vi "AttackerStop.vi"(6 "atacando contra?":bool, 8 "IA State Input 2":T1, 9 "balls":T5[](array[typedef]), 10 "Field Size in":T6, 11 "Robot in":T2={"id"=0, "function"=enum."Attacker", "x"=0.0, "y"=0.0, "orientation"=0.0, "v_tangent"=0.0, "v_normal"=0.0, "v_ang"=0.0, "kick_x"=0.0, "kick_z"=0.0, "dribble"=FALSE, "Timestamp"=timestamp(0 s since 1904-01-01), "dest_x"=0.0, "dest_y"=0.0, "dest_orientation"=0.0, "estimatives"={"est_v_tangent"=0.0, "est_v_normal"=0.0, "est_vx"=0.0, "est_vy"=0.0}, "dest_x_kick"=0.0, "dest_y_kick"=0.0, "Gap Coord"=[], "States"=enum."GoToTangent"}) -> (3 "Robot out":T2={"id"=0, "function"=enum."Attacker", "x"=0.0, "y"=0.0, "orientation"=0.0, "v_tangent"=0.0, "v_normal"=0.0, "v_ang"=0.0, "kick_x"=0.0, "kick_z"=0.0, "dribble"=FALSE, "Timestamp"=timestamp(0 s since 1904-01-01), "dest_x"=0.0, "dest_y"=0.0, "dest_orientation"=0.0, "estimatives"={"est_v_tangent"=0.0, "est_v_normal"=0.0, "est_vx"=0.0, "est_vy"=0.0}, "dest_x_kick"=0.0, "dest_y_kick"=0.0, "Gap Coord"=[], "States"=enum."GoToTangent"})   [LabVIEW 2016]
uses:
  Core/Field Size.ctl
  Core/AI Robot.ctl
  Functions Enum.ctl
  AttackerStates.ctl
  Core/AI Ball.ctl
  Core/AI Input.ctl
  Core/AI Judge.ctl
  Command Enum.ctl
  Util/Events/Events.ctl
  <vilib>/Analysis/_algsub.llb/Real Vector Norm.vi
  <vilib>/Analysis/NI_AALPro.lvlib
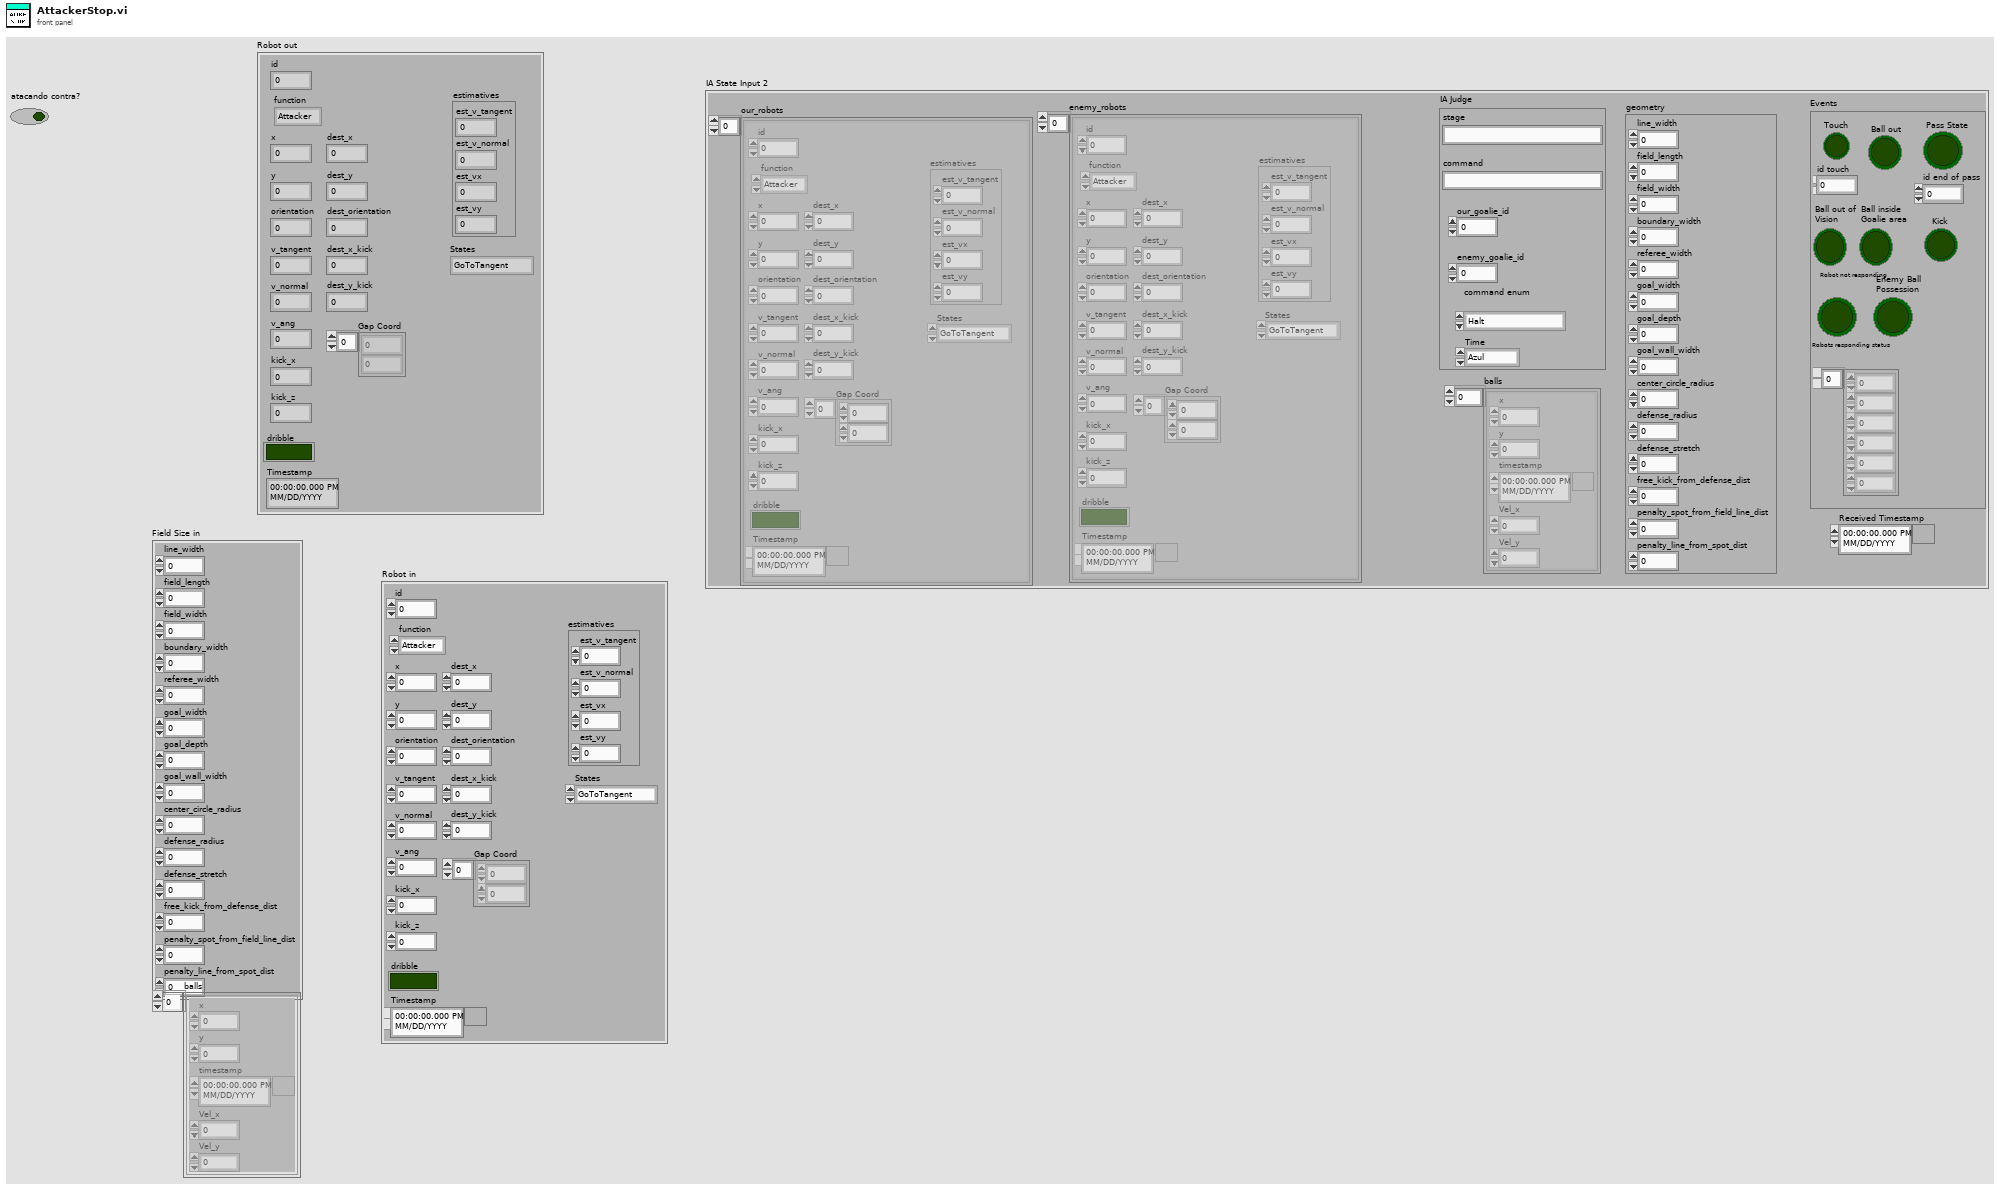
[diagram p1: front panel]
types:
  T1 = typedef "AI Input.ctl" = cluster{"our_robots":T2[], "enemy_robots":T2[], "balls":T5[], "geometry":T6, "IA Judge":T7, "Received Timestamp":timestamp, "Events":T9}
  T2 = typedef "AI Robot.ctl" = cluster{"id":u32, "function":T3, "x":dbl, "y":dbl, "orientation":dbl, "v_tangent":dbl, "v_normal":dbl, "v_ang":dbl, "kick_x":dbl, "kick_z":dbl, "dribble":bool, "Timestamp":timestamp, "dest_x":dbl, "dest_y":dbl, "dest_orientation":dbl, "estimatives":cluster{"est_v_tangent":dbl, "est_v_normal":dbl, "est_vx":dbl, "est_vy":dbl}, "dest_x_kick":dbl, "dest_y_kick":dbl, "Gap Coord":dbl[], "States":T4}
  T3 = typedef "Functions Enum.ctl" = enum16{"Attacker", "Goalie", "Defender", "Striker", "Goto 0", "Dummy", "Kicker", "ZigZag"}
  T4 = typedef "AttackerStates.ctl" = enum16{"Pass", "GoToTangent", "BallGetting", "GoToKick", ""}
  T5 = typedef "AI Ball.ctl" = cluster{"x":dbl, "y":dbl, "timestamp":timestamp, "Vel_x":dbl, "Vel_y":dbl}
  T6 = typedef "Field Size.ctl" = cluster{"line_width":u32, "field_length":u32, "field_width":u32, "boundary_width":u32, "referee_width":u32, "goal_width":u32, "goal_depth":u32, "goal_wall_width":u32, "center_circle_radius":u32, "defense_radius":u32, "defense_stretch":u32, "free_kick_from_defense_dist":u32, "penalty_spot_from_field_line_dist":u32, "penalty_line_from_spot_dist":u32}
  T7 = typedef "AI Judge.ctl" = cluster{"stage":string, "command":string, "our_goalie_id":dbl, "enemy_goalie_id":dbl, "command enum":T8, "Time":enum16{"Azul", "Amarelo"}}
  T8 = typedef "Command Enum.ctl" = enum16{"Halt", "Stop", "Force Start", "PKA Normal Start", "Prepare Kickoff Ally", "PKE Normal Start", "Prepare Kickoff Enemy", "Prepare Penalty Ally", "PPA Normal Start", "Prepare Penalty Enemy", "PPE Normal Start", "Direct Free Enemy", "Direct Free Ally", "Indirect Free Enemy", "Indirect Free Ally", "Timeout Enemy", "Timeout Ally", "Goal Enemy", "Goal Ally", "Ball Placement Enemy", "Ball Placement Ally", "Normal Half Time", "Extra Time Break", "Extra Half Time", "None"}
  T9 = typedef "Events.ctl" = cluster{"Touch":bool, "Ball out":bool, "id touch":dbl, "Ball out of \nVision":bool, "Ball inside \nGoalie area":bool, "Robot not responding":bool, "Robots responding status":dbl[], "Enemy Ball \nPossession":bool, "Pass State":bool, "id end of pass":dbl, "Kick":bool}
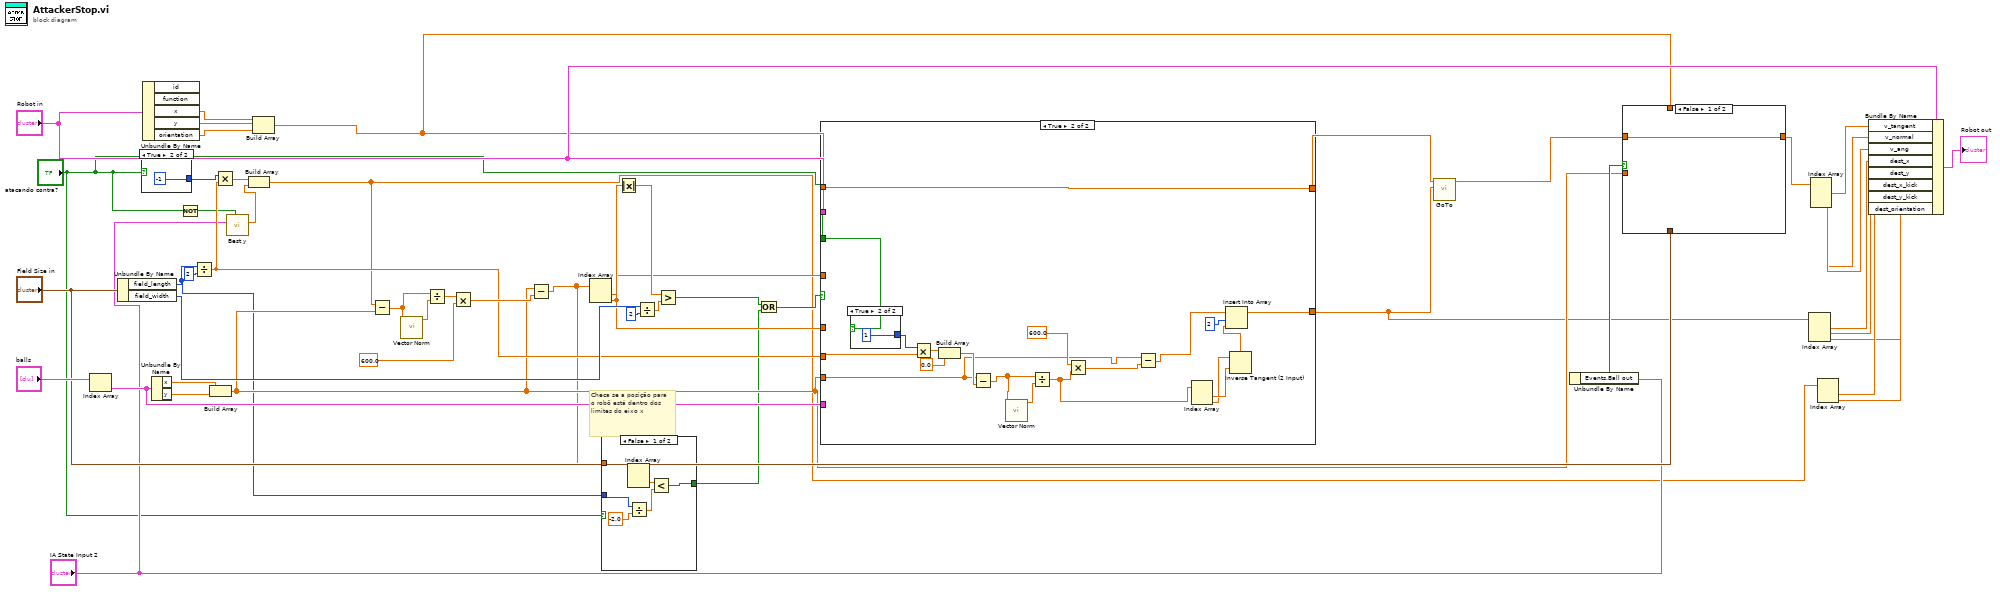
[diagram p0: block diagram]
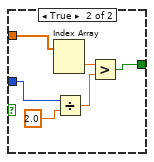
[diagram p2: hidden frame]
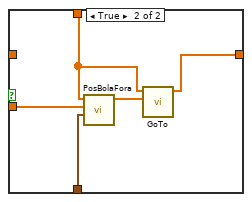
[diagram p3: hidden frame]
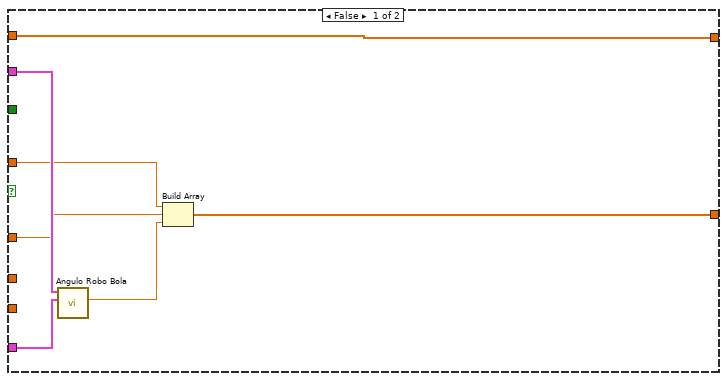
[diagram p4: hidden frame]
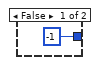
[diagram p5: hidden frame]
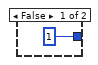
[diagram p6: hidden frame]
diagram:
  # "Checa se a posição para o robõ está dentro dos limites do eixo x"
  n1 = Index Array(array="balls") -> (element=w37:T5)  [unwired: 1 in]
  n2 = Unbundle By Name("Field Size in") -> ("field_length"=w14:u32, "field_width"=w39:u32)
  n3 = case shown="True" "atacando contra?" {
    tunnel: [1 -1] -> w48
    frame False {
    }
    frame True {
    }
  }
  n4 = Unbundle By Name("Robot in") -> ("x"=w34:dbl, "y"=w33:dbl, "orientation"=w32:dbl)  [unwired: 2 out]
  n5 = Unbundle By Name(w37) -> ("x"=w47:dbl, "y"=w46:dbl)
  n6 = Not(x="atacando contra?") -> (.not. x?=w6:bool)
  n7 = Divide(x=w14, y=u32 2) -> (x/y=w17:dbl)
  n8 = Build Array(w47, w46) -> (w16:dbl[])
  n9 = Multiply(x=w48, y=w17) -> (x*y=w45:dbl)
  n10 = call "Best y.vi"("inimigos"=w6, "IA State"="IA State Input 2") -> ("Best y"=w7:dbl)  [unwired: 6 in, 3 out]
  n11 = Build Array(w45, w7) -> (w4:dbl[])
  n12 = Build Array(w34, w33, w32) -> (w23:dbl[])
  n13 = Subtract(x=w4, y=w16) -> (x-y=w44:dbl[])
  n14 = call-poly <vilib>:"Vector Norm.vi"("Input Vector"=w44) -> ("norm"=w43:dbl)  [unwired: 9 in, 1 out]
  n15 = Divide(x=w44, y=w43) -> (x/y=w42:dbl[])
  n16 = Multiply(x=w42, y=600.0) -> (x*y=w20:dbl[])
  n17 = Subtract(x=w16, y=w20) -> (x-y=w15:dbl[])
  n18 = Index Array(array=w15) -> (element #1=w35:dbl, element #2=w36:dbl)  [unwired: 2 in]
  n19 = case shown="False" "atacando contra?" {
    tunnel: w14 -> [w56 w62]
    tunnel: [w55 w59] -> w9
    tunnel: w15 -> [w54 w63]
    frame False {
      n20 = Index Array(array=w54) -> (element #1=w58:dbl)  [unwired: 2 in, 1 out]
      n21 = Divide(x=w56, y=-2.0) -> (x/y=w57:dbl)
      n22 = Less?(x=w58, y=w57) -> (x < y?=w55:bool)
    }
    frame True {
      n23 = Index Array(array=w63) -> (element #1=w61:dbl)  [unwired: 2 in, 1 out]
      n24 = Divide(x=w62, y=2.0) -> (x/y=w60:dbl)
      n25 = Greater?(x=w61, y=w60) -> (0:w59:bool)
    }
  }
  n26 = Absolute Value(x=w36) -> (abs(x)=w41:dbl)
  n27 = Divide(x=w39, y=u32 2) -> (x/y=w38:dbl)
  n28 = Greater?(x=w41, y=w38) -> (0:w10:bool)
  n29 = Or(x=w10, y=w9) -> (x .or. y?=w11:bool)
  n30 = case shown="True" w11 {
    tunnel: w37 -> [w71 _]
    tunnel: "Robot in" -> [w70 _]
    tunnel: w36 -> [w68 _]
    tunnel: w35 -> [w67 _]
    tunnel: w23 -> [w66 w77]
    tunnel: w16 -> [_ w73]
    tunnel: "atacando contra?" -> [_ w84]
    tunnel: w17 -> [_ w89]
    tunnel: [w66 w77] -> w13
    tunnel: [w65 w76] -> w12
    frame False {
      n31 = call "Angulo Robo Bola.vi"("Ball"=w71, "Robot"=w70) -> ("Angulo"=w69:dbl)  [unwired: 9 in]
      n32 = Build Array(w67, w68, w69) -> (w65:dbl[])
    }
    frame True {
      n33 = case shown="True" w84 {
        tunnel: [-1 1] -> w90
        frame False {
        }
        frame True {
        }
      }
      n34 = Multiply(x=w90, y=w89) -> (x*y=w88:dbl)
      n35 = Build Array(w88, 0.0 ("element")) -> (w83:dbl[])
      n36 = Subtract(x=w73, y=w83) -> (x-y=w85:dbl[])
      n37 = call-poly <vilib>:"Vector Norm.vi"("Input Vector"=w85) -> ("norm"=w86:dbl)  [unwired: 9 in, 1 out]
      n38 = Divide(x=w85, y=w86) -> (x/y=w78:dbl[])
      n39 = Multiply(x=600.0, y=w78) -> (x*y=w74:dbl[])
      n40 = Subtract(x=w73, y=w74) -> (x-y=w72:dbl[])
      n41 = Index Array(array=w78) -> (element #1=w80:dbl, element #2=w79:dbl)  [unwired: 2 in]
      n42 = Inverse Tangent (2 Input)(1:w80, 2:w79) -> (0:w81:dbl)
      n43 = Insert Into Array(array=w72, index=2, new element=w81) -> (w76:dbl[])
    }
  }
  n44 = call "GoTo.vi"("Target"=w12, "Position"=w13) -> ("Output\nVelocity"=w22:dbl[])  [unwired: 8 in, 1 out]
  n45 = Unbundle By Name("IA State Input 2") -> ("Events.Ball out"=w31:bool)
  n46 = case shown="False" w31 {
    tunnel: w22 -> [w93 _]
    tunnel: [w93 w94] -> w25
    tunnel: "Field Size in" -> [_ w98]
    tunnel: w23 -> [_ w95]
    tunnel: w16 -> [_ w97]
    frame False {
    }
    frame True {
      n47 = call "PosBolaFora.vi"("Field Size in"=w98, "Position da bola"=w97, "Position do robot"=w95) -> ("Target"=w96:dbl[])  [unwired: 8 in]
      n48 = call "GoTo.vi"("Target"=w96, "Position"=w95) -> ("Output\nVelocity"=w94:dbl[])  [unwired: 8 in, 1 out]
    }
  }
  n49 = Index Array(array=w12) -> (element #1=w19:dbl, element #2=w18:dbl, element #3=w1:dbl)  [unwired: 3 in]
  n50 = Index Array(array=w25) -> (element #1=w28:dbl, element #2=w29:dbl, element #3=w30:dbl)  [unwired: 3 in]
  n51 = Index Array(array=w4) -> (element #1=w3:dbl, element #2=w2:dbl)  [unwired: 2 in]
  n52 = Bundle By Name(cluster="Robot in", "v_tangent"=w28, "v_normal"=w29, "v_ang"=w30, "dest_x"=w19, "dest_y"=w18, "dest_x_kick"=w3, "dest_y_kick"=w2, "dest_orientation"=w1) -> (→"Robot out":T2)
